vi "niFPGA BFGroup Input Buffer 4096 U64.vi"(0 "data in":u64=8, 1 "reset":bool) -> (4 "x out":u64, 6 "y out":u64)   [LabVIEW 2017]
uses:
  <vilib>/Utility/error.llb/Clear Errors.vi
  <vilib>/rvi/Emulation/niFpgaSctlEmulationGetInTimedLoop.vi
  <vilib>/rvi/DataTransferAndStorage/Container/Common/niFpgaContainerGetUniqueNameForEmu.vi
  <vilib>/rvi/DataTransferAndStorage/Container/Common/niFpgaContainerSetEmuInfo.vi
  <vilib>/rvi/eio/common/nirviEmuReportErrorAndStop.vi
  <vilib>/rvi/Memory/Memory_Emulation/nirvimemoryEmulation.vi
  <vilib>/rvi/Memory/Memory_Emulation/nirvimemoryFastEmulation.vi
  <vilib>/rvi/Memory/Memory_Emulation/niFpgaMemoryEmulationCacheClearOnFirstRun.vi
  <vilib>/rvi/Memory/Memory_Emulation/nirvimemoryEmulationManagerCache_MakeExclusive.vi
  <vilib>/rvi/Memory/Memory_Emulation/niFpgaMemoryEmulationValidateCache.vi
  <vilib>/rvi/Memory/Memory_Emulation/nirvimemoryEmulationManagerCache_InsertValue.vi
  <vilib>/rvi/Memory/Memory_Emulation/nirvimemoryEmulationManagerCache_ReleaseExclusive.vi
  <vilib>/rvi/Memory/Memory_Emulation/nirvimemoryEmulationManagerCache_GetValue.vi
  <vilib>/rvi/Emulation/niFpgaEmulationIsFPGAContextNoSignature.vi
  <vilib>/rvi/Memory/Memory_Emulation/nirvimemoryEmulationManagerCache_SetValue.vi
  <vilib>/rvi/Emulation/niFpgaSctlEmulationResourceMgr.vi
  <vilib>/rvi/LocalResourceManager/LocalResourceManager.xnode
  <vilib>/rvi/DataTransferAndStorage/Container/XNode/niFpgaContainer.xnode
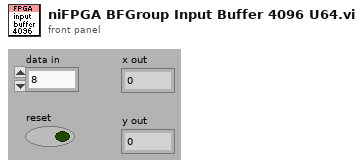
[diagram p1: front panel]
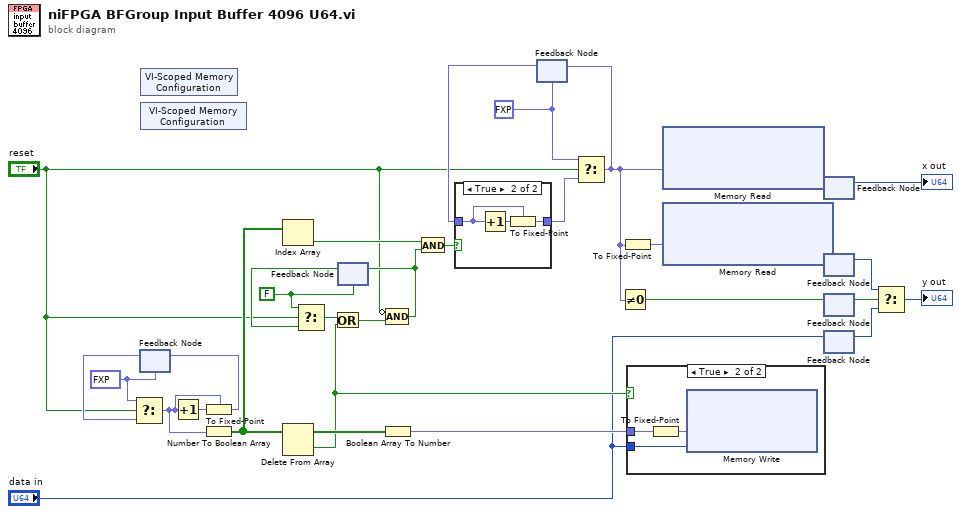
[diagram p0: block diagram]
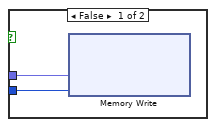
[diagram p3: hidden frame]
diagram:
  w21 = fxp<+,11,11> 0.0
  w14 = FALSE
  w25 = fxp<+,12,12> 4095.0
  n1 = feedback #1(w25) -> (w31:fxp<+,12,12>)
  n2 = Select(t=w25, s="reset", f=w31) -> (s? t:f=w9:fxp<+,12,12>)
  n3 = xnode "VI-Scoped Memory Configuration"() -> ()  [unwired: 1 out]
  n4 = xnode "VI-Scoped Memory Configuration"() -> ()  [unwired: 1 out]
  n5 = Increment(x=w9) -> (x+1=w11:fxp<+,13,13>)
  n6 = To Fixed-Point(fixed-point type=w9, number=w11) -> (fixed-point=w10:fxp<+,12,12>)
  n7 = feedback-in #1(w10) -> ()
  n8 = Number To Boolean Array(number=w9) -> (Boolean array=w26:bool[])
  n9 = Index Array(array=w26) -> (element=w30:bool)  [unwired: 1 in]
  n10 = Delete From Array(array=w26) -> (deleted portion=w28:bool, array with subset deleted=w29:bool[])  [unwired: 2 in]
  n11 = feedback #2(w14) -> (w8:bool)
  n12 = Select(t=w14, s="reset", f=w8) -> (s? t:f=w15:bool)
  n13 = Or(x=w15, y=w28) -> (x .or. y?=w13:bool)
  n14 = Boolean Array To Number(Boolean array=w29) -> (number=w27:fxp<+,11,11>)
  n15 = Compound Arithmetic op=AND(invert "reset", w13) -> (w12:bool)
  n16 = feedback-in #2(w12) -> ()
  n17 = And(x=w30, y=w12) -> (x .and. y?=w22:bool)
  n18 = feedback #3(w21) -> (w24:fxp<+,11,11>)
  n19 = case shown="True" w22 {
    tunnel: w24 -> [w32 w33]
    tunnel: [w32 w34] -> w23
    frame False {
    }
    frame True {
      n20 = Increment(x=w33) -> (x+1=w35:fxp<+,12,12>)
      n21 = To Fixed-Point(fixed-point type=w33, number=w35) -> (fixed-point=w34:fxp<+,11,11>)
    }
  }
  n22 = Select(t=w21, s="reset", f=w23) -> (s? t:f=w6:fxp<+,11,11>)
  n23 = feedback-in #3(w6) -> ()
  n24 = Not Equal To 0?(x=w6) -> (x != 0?=w5:bool)
  n25 = To Fixed-Point(number=w6) -> (fixed-point=w16:fxp<+,10,10>)  [unwired: 1 out]
  n26 = case shown="True" w28 {
    tunnel: "data in" -> [w37 w40]
    tunnel: w27 -> [w36 w39]
    frame False {
      n27 = xnode ("Memory Write")("Address"=w36, "Data"=w37) -> ()  [unwired: 2 out]
    }
    frame True {
      n28 = To Fixed-Point(number=w39) -> (fixed-point=w38:fxp<+,10,10>)  [unwired: 1 out]
      n29 = xnode ("Memory Write")("Address"=w38, "Data"=w40) -> ()  [unwired: 2 out]
    }
  }
  n30 = xnode ("Memory Read")("Address"=w6) -> ("Data"=w20:u64)  [unwired: 2 out]
  n31 = xnode ("Memory Read")("Address"=w16) -> ("Data"=w17:u64)  [unwired: 2 out]
  n32 = feedback-in #4(w20) -> ()
  n33 = feedback #4() -> (→"x out":u64)  [unwired: 1 out]
  n34 = feedback-in #5(w17) -> ()
  n35 = feedback #5() -> (w2:u64)  [unwired: 1 out]
  n36 = feedback-in #6(w5) -> ()
  n37 = feedback #6() -> (w4:bool)  [unwired: 1 out]
  n38 = feedback-in #7("data in") -> ()
  n39 = feedback #7() -> (w3:u64)  [unwired: 1 out]
  n40 = Select(t=w2, s=w4, f=w3) -> (s? t:f=→"y out":u64)
